vi "托盘料满状态判断.vi"(9 "有空料？":bool, 10 "全盘料满？":bool, 11 "托盘料满？":bool) -> (1 "OK？":bool, 2 "数值":i32)   [LabVIEW 2014]
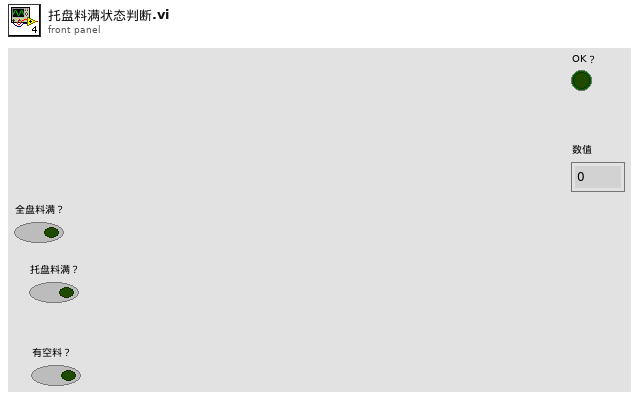
[diagram p1: front panel]
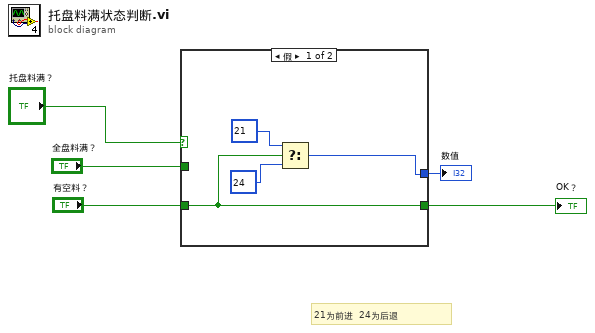
[diagram p0: block diagram]
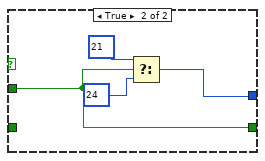
[diagram p2: hidden frame]
diagram:
  # "21为前进  24为后退"
  n1 = case shown="假" "托盘料满？" {
    tunnel: "全盘料满？" -> [_ w10]
    tunnel: [w7 w11] -> w2
    tunnel: "有空料？" -> [w6 _]
    tunnel: [w6 w10] -> w1
    frame False {
      n2 = Select(t=21, s=w6, f=24) -> (s? t:f=w7:i32)
    }
    frame True {
      n3 = Select(t=21, s=w10, f=24) -> (s? t:f=w11:i32)
    }
  }
  "数值" <- w2
  "OK？" <- w1
